vi "AccelCtrl.vi"(8 "CurrentSpeed":dbl, 11 "TargetSpeed":dbl) -> (2 "Speed":dbl)   [LabVIEW 2015]
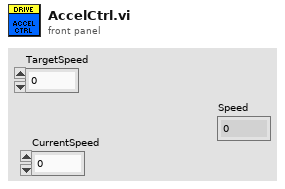
[diagram p1: front panel]
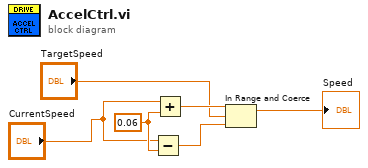
[diagram p0: block diagram]
diagram:
  w6 = 0.06 ("y")
  n1 = Subtract(x="CurrentSpeed", y=w6) -> (x-y=w4:dbl)
  n2 = Add(x="CurrentSpeed", y=w6) -> (x+y=w5:dbl)
  n3 = In Range and Coerce(upper limit=w5, x="TargetSpeed", lower limit=w4) -> (coerced(x)=→"Speed":dbl)  [unwired: 1 out]
